vi "Document My VI - Describe My VI.vi"(8 "error in (no error)":errorcluster, 9 "Config Data":cluster{"Company":string, "Author":string}={"Company"="Good Automation, LLC", "Author"="Your Name Here"}, 11 "Active VI Ref In":refnum<vi>) -> (0 "error out":errorcluster, 3 "Active VI Ref Out":refnum<vi>)   [LabVIEW 2014]
uses:
  TYPE_Version Status.ctl
  TYPE_Description Cluster.ctl
  <vilib>/Utility/miscctls.llb/LVBoundsTypeDef.ctl
  <vilib>/regexp/Match Regular Expression.xnode
panel:
  in  "Requirement Coverage":string[](array[string])
  in  "Bold Text":bool
  in  "Copy Desc":bool
  in  "VI Description":string caption="Enter The Text To Provide A Functional Description Of The VI"
  in  "Cancel Button":bool
  out "VI's New Description":string
  out "Icon":picture
  in  "Set No Review":bool
  in  "Use Today":bool
  in  "Date of Review":timestamp=timestamp(3345454800 s since 1904-01-01) format="%<%m/%d/%Y>T"
  in  "Index":u32=1 min=1
  in  "Minor":u16 caption="Major"
  in  "Major":u16 min=1
  in  "Status":T1
  out "Copyright":string
  out "Author(s)":string
  out "VI's Original Description":string
  in  "Save":bool
  # "."
  # "."
  # "Functional Description"
  # "Version Information"
  # "Autoset Information"
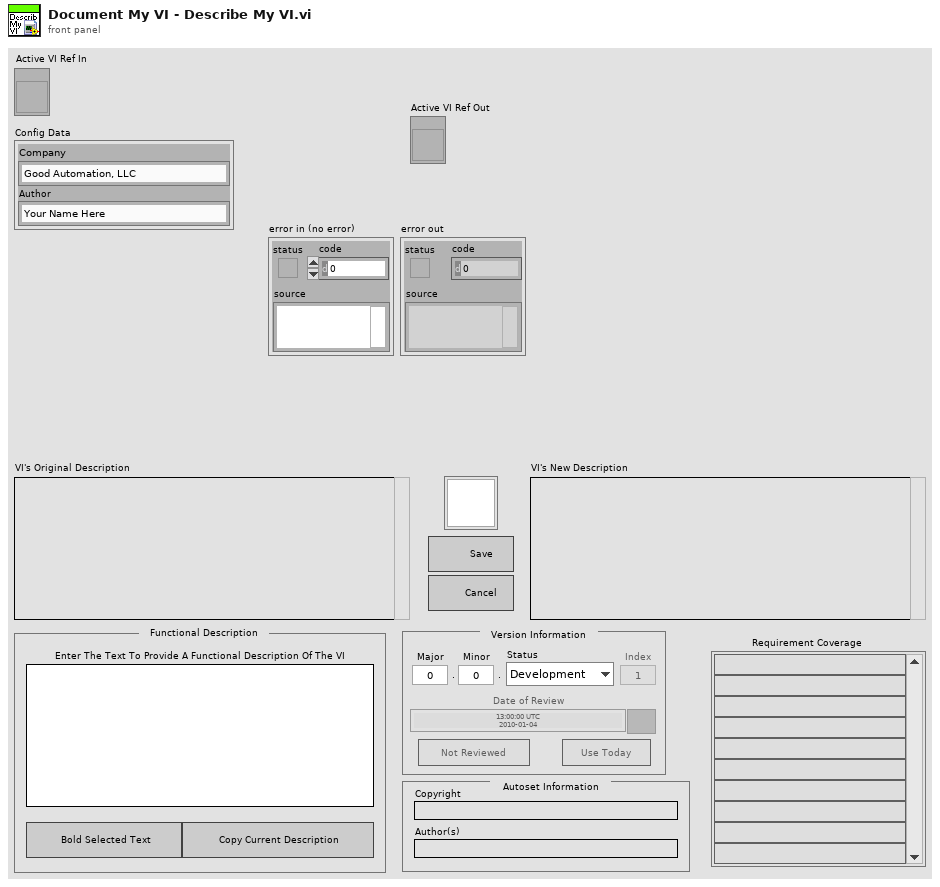
[diagram p1: front panel]
types:
  T1 = typedef "TYPE_Version Status.ctl" = enum16{"Development", "alpha", "beta", "Reviewed", "Bug", "Other"}
  T2 = enum32{"invalid app kind", "Development System", "Run Time System", "Student Edition", "Embedded LabVIEW", "Evaluation", "Custom"}
  T3 = enum8{"Enabled", "Disabled", "Disabled and Grayed Out"}
  T4 = enum32{"Invalid", "Standard", "Closed", "Hidden", "Minimized", "Maximized"}
  T5 = typedef "LVBoundsTypeDef.ctl" = cluster{"Width":u32, "Height":u32}
  T6 = typedef "TYPE_Description Cluster.ctl" = cluster{"VI Description":string, "VI Version":string, "Review Date":string, "Author":string, "Copyright":string, "Requirements Coverage":string}
  T7 = cluster{"Core":cluster{"Current VI Reference":refnum<vi>, "Close Panel on Exit?":bool}, "Config Data":cluster{"Company":string, "Author":string}, "Active VI Ref In":refnum<vi>, "Description":T6, "Original Description":string}
  T8 = cluster{"Current VI Reference":refnum<vi>, "Close Panel on Exit?":bool}
  T9 = typedef "imagedata.ctl" = cluster{"image type":i32, "image depth":i32, "image":u8[], "mask":u8[], "colors":u32[], "Rectangle":cluster{"left":i16, "top":i16, "right":i16, "bottom":i16}}
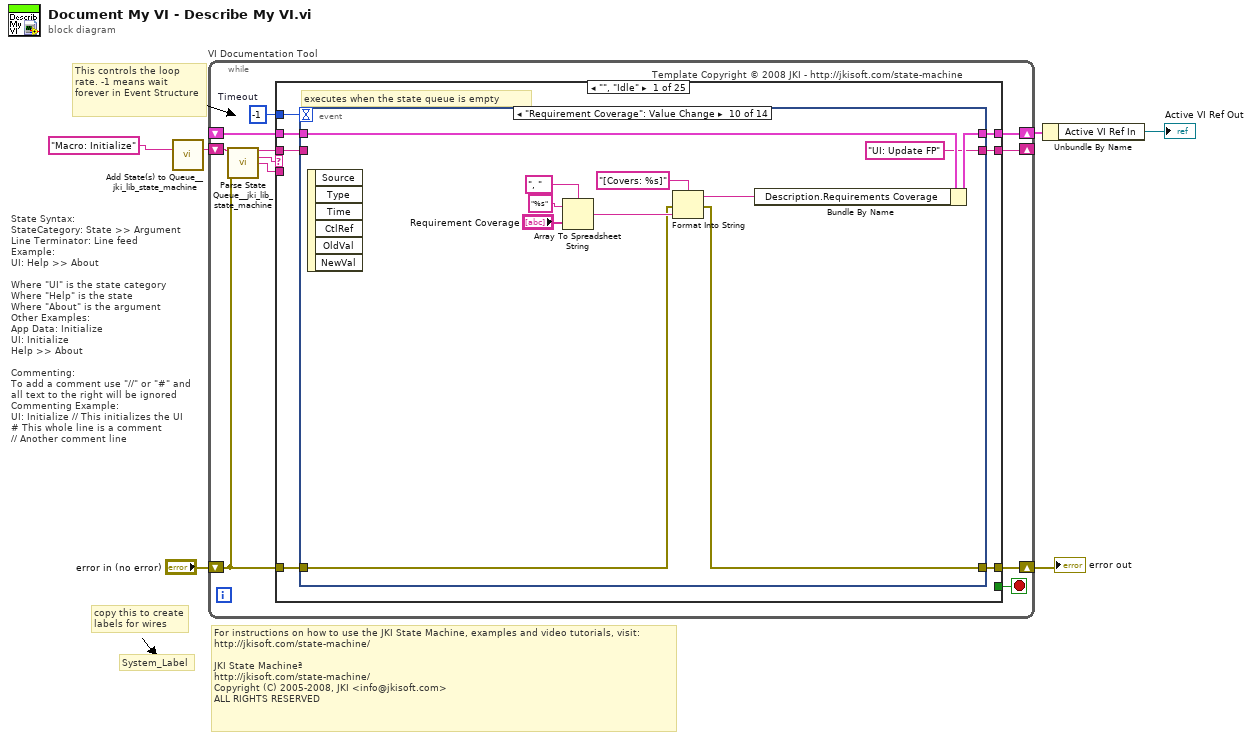
[diagram p0: block diagram]
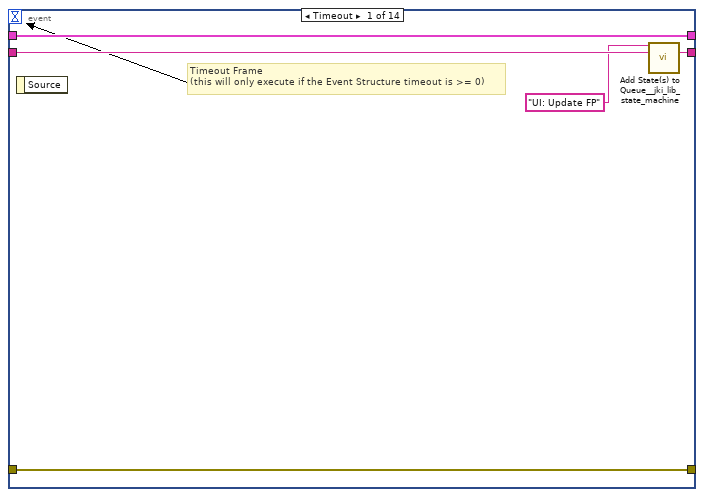
[diagram p2: hidden frame]
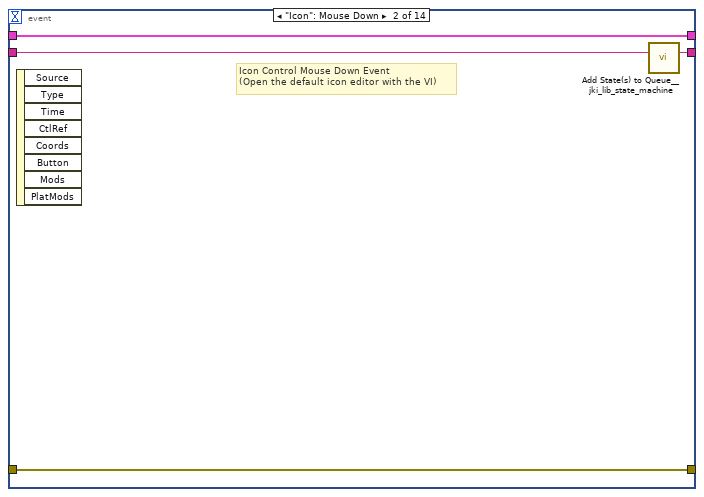
[diagram p3: hidden frame]
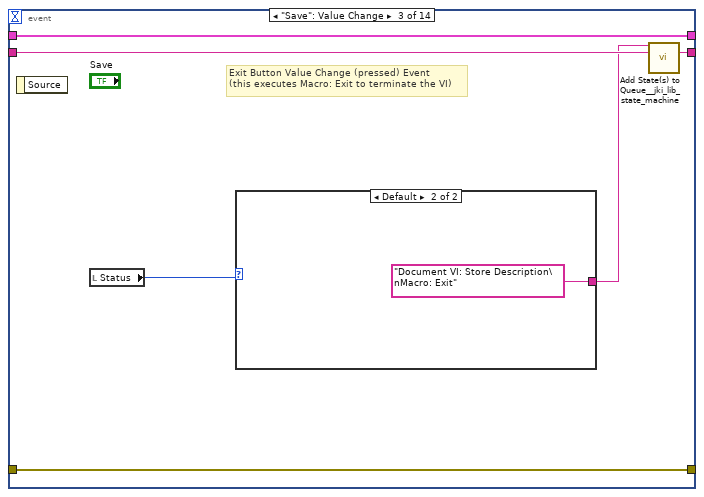
[diagram p4: hidden frame]
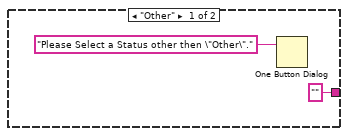
[diagram p5: hidden frame]
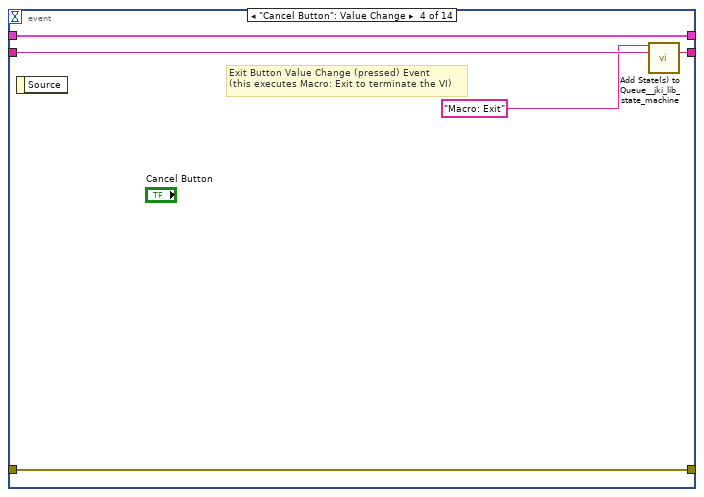
[diagram p6: hidden frame]
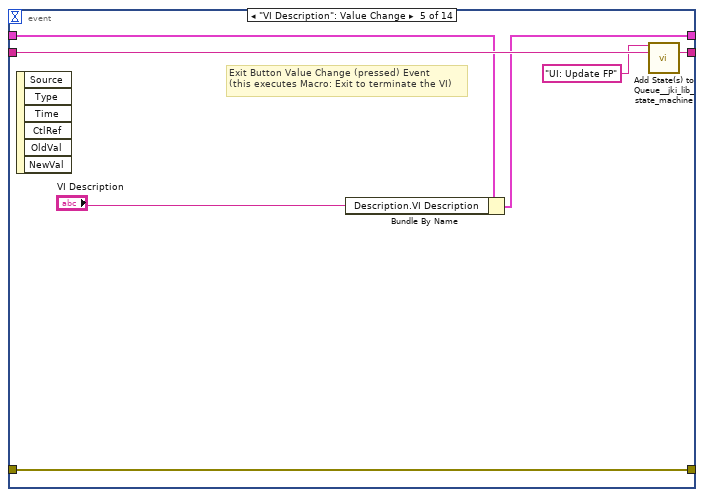
[diagram p7: hidden frame]
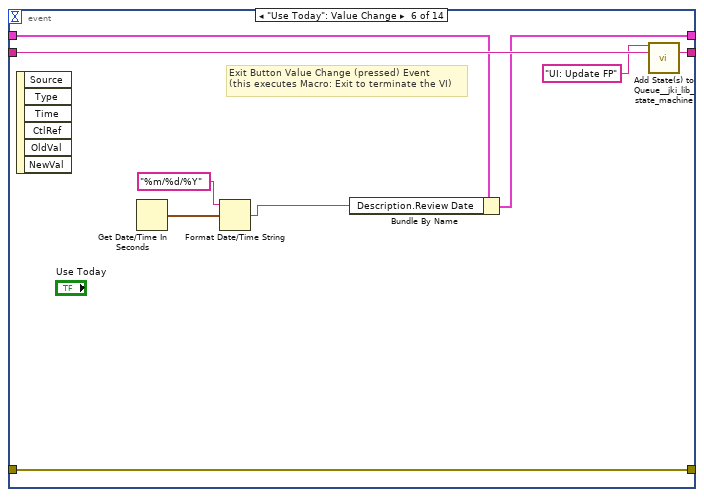
[diagram p8: hidden frame]
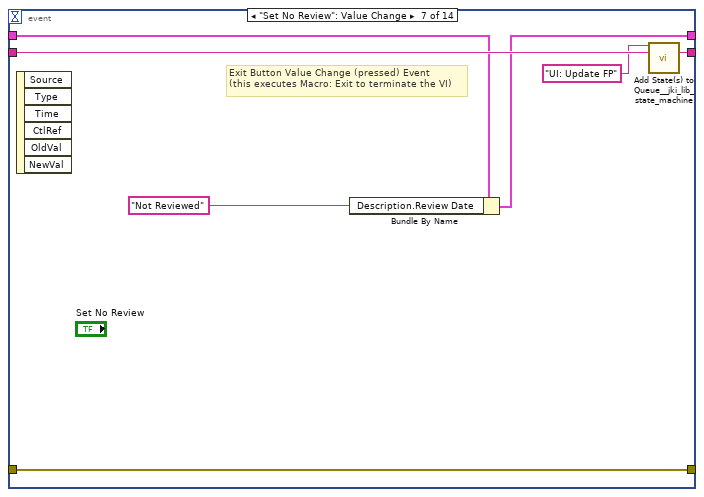
[diagram p9: hidden frame]
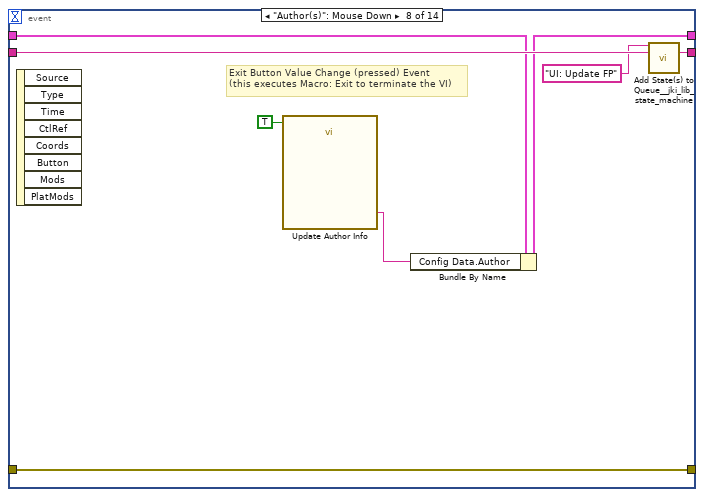
[diagram p10: hidden frame]
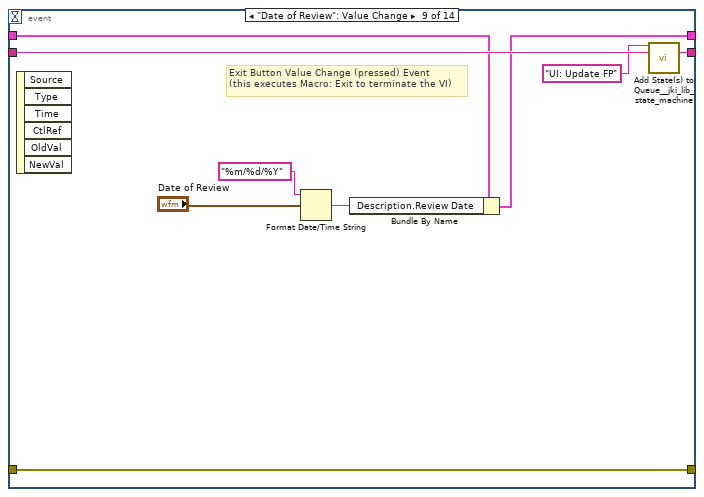
[diagram p11: hidden frame]
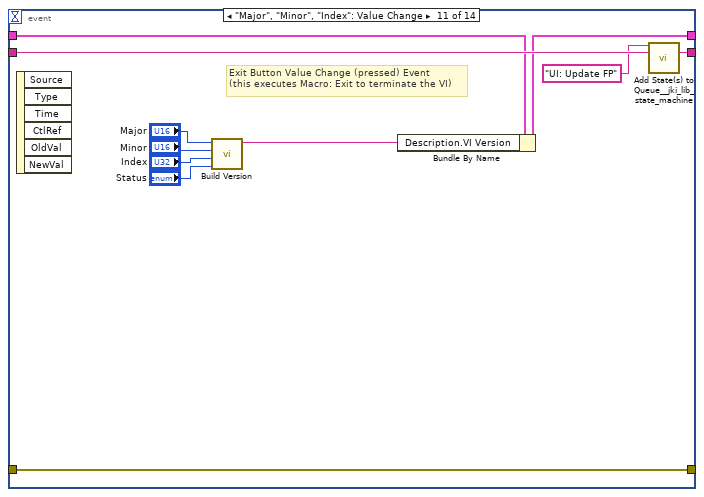
[diagram p12: hidden frame]
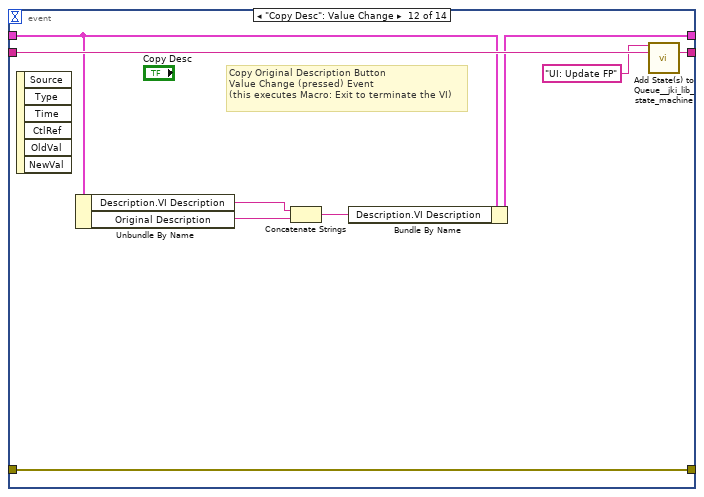
[diagram p13: hidden frame]
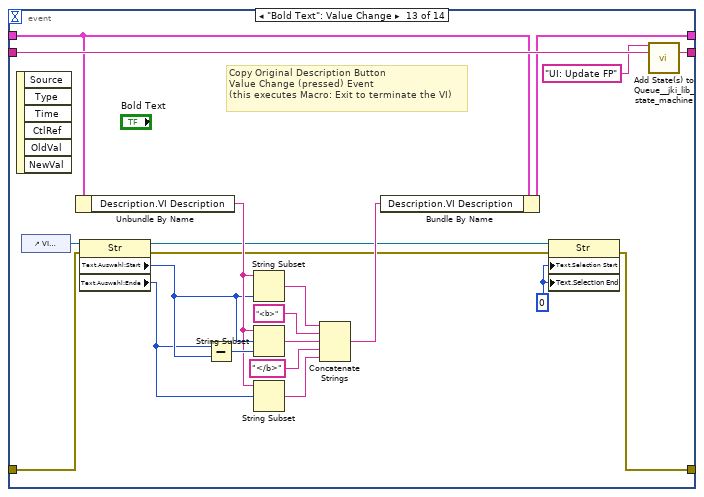
[diagram p14: hidden frame]
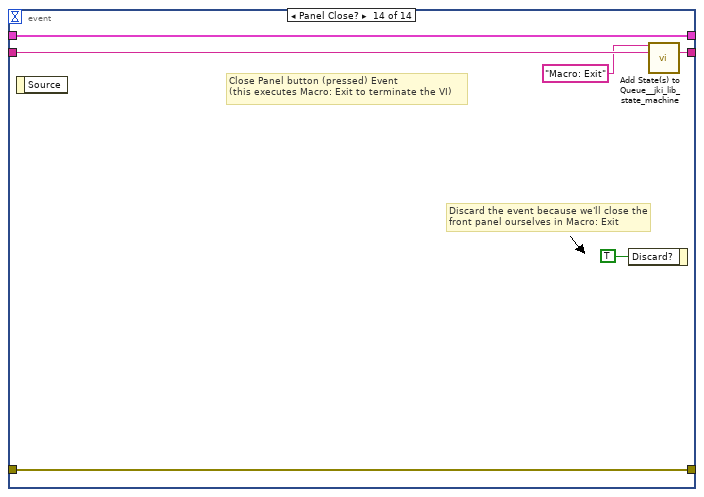
[diagram p15: hidden frame]
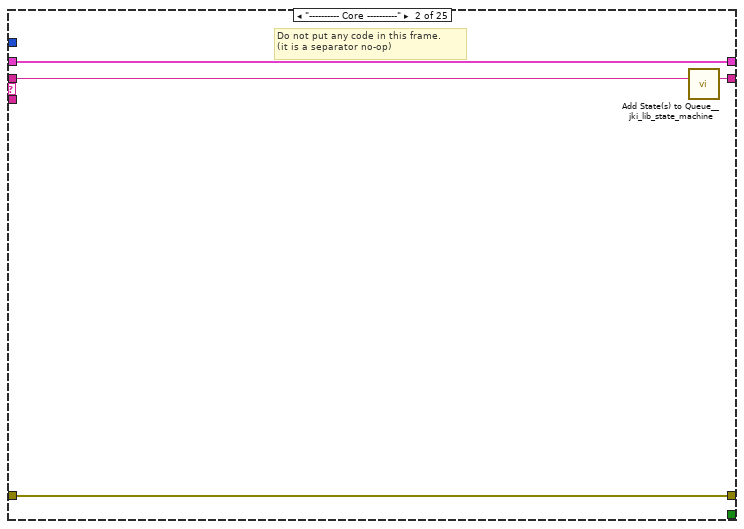
[diagram p16: hidden frame]
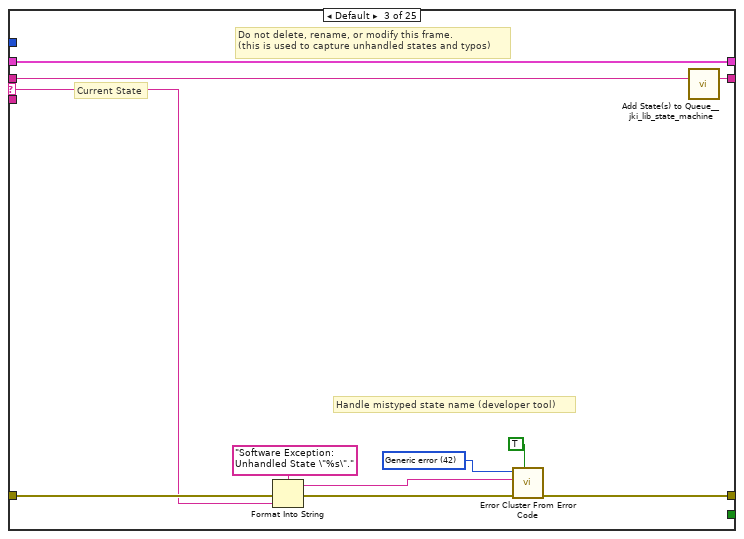
[diagram p17: hidden frame]
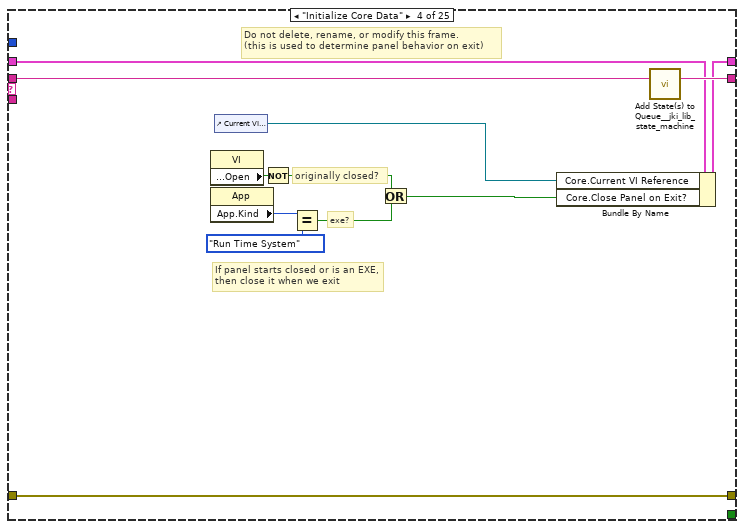
[diagram p18: hidden frame]
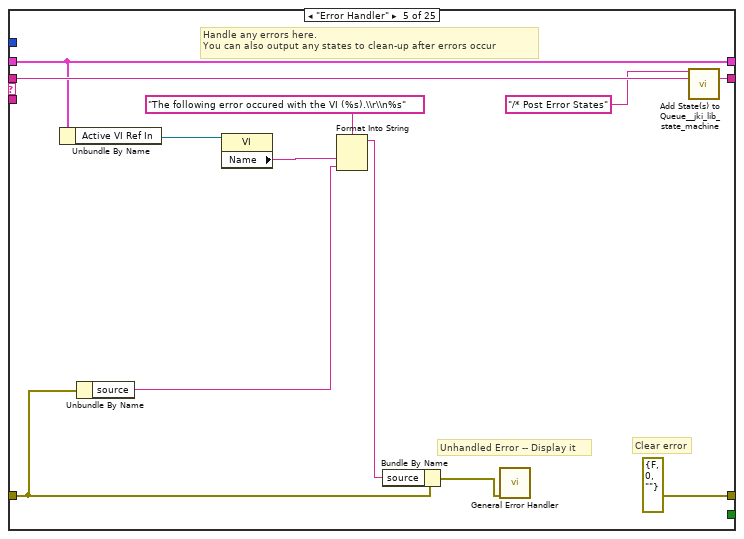
[diagram p19: hidden frame]
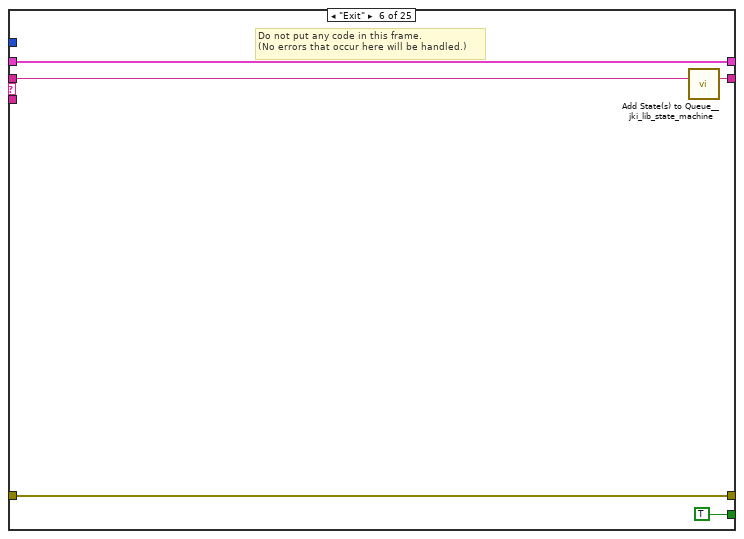
[diagram p20: hidden frame]
diagram:
  # "This controls the loop rate. -1 means wait forever in Event Structure"
  # "For instructions on how to use the JKI State Machine, examples and video tutorials, visit:\nhttp://jkisoft.com/state-machine/\n\nJKI State Machineª\nhttp://jkisoft.com/state-machine/\nCopyright (C) 2005-2008, JKI <info@jkisoft.com>\nALL RIGHTS RESERVED"
  # "State Syntax:\nStateCategory: State >> Argument\nLine Terminator: Line feed\nExample:\nUI: Help >> About\n\nWhere \"UI\" is the state category\nWhere \"Help\" is the state\nWhere \"About\" is the argument\nOther Examples:\nApp Data: Initialize\nUI: Initialize\nHelp >> About\n\nCommenting:\nTo add a comment use \"//\" or \"#\" and all text to the right will be ignored\nCommenting Example:\nUI: Initialize // This initializes the UI\n# This whole line is a comment\n// Another comment line"
  # "copy this to create labels for wires"
  # "System_Label"
  n1 = call <vilib>:"Add State(s) to Queue__jki_lib_state_machine.vi"("State(s) in (\"\")"="Macro: Initialize") -> ("States Out"=w6:string)  [unwired: 14 in]
  n2 = while "VI Documentation Tool" {
    shift-right: [w10] -> w2
    shift-left: _ -> [w9]
    shift-right: [w13] -> w3
    shift-left: "error in (no error)" -> [w7]
    shift-right: [w12] -> _
    shift-left: w6 -> [w14]
    stop <- w11 stop-if-true
    w8 = -1  # Timeout
    # "Template Copyright © 2008 JKI - http://jkisoft.com/state-machine"
    n3 = call <vilib>:"Parse State Queue__jki_lib_state_machine.vi"("State Queue"=w14, "Error In (no error)"=w7) -> ("Remaining States"=w16:string, "Current State"=w17:string, "Arguments"=w15:string)  [unwired: 11 in]
    n4 = case shown="\"\", \"Idle\"" w17 {
      selector: w17 -> [_ _ w150 _ _ _ _ _ _ _ _ _ _ _ _ _ _ _ _ _ _ _ _ _ _]
      tunnel: w16 -> [w24 w149 w154 w172 w184 w189 w193 w202 w208 w212 w218 w245 w372 w393 w404 w430 w435 w445 w450 w455 w459 w475 w489 w504 w517]
      tunnel: w15 -> [_ _ _ _ _ _ _ _ _ _ _ _ _ w388 w398 _ _ _ _ _ _ _ _ _ _]
      tunnel: w9 -> [w22 w146 w152 w163 w179 w187 w190 _ w203 w209 w214 w242 w369 w391 w400 w427 w432 w442 w447 w452 w456 w472 w484 w502 w515]
      tunnel: [w21 w147 w156 w169 errorcluster {"status"=FALSE, "code"=0, "source"=""} ("error out") w186 w191 w199 w204 w210 w215 w243 w370 w389 w401 w428 w433 w443 w448 w453 w457 w468 w479 w500 w513] -> w13
      tunnel: w7 -> [w20 w147 w155 w169 w178 w186 w191 w199 w205 w210 w216 w243 w370 w390 w402 w428 w433 w443 w448 w453 w457 w470 w482 w500 w513]
      tunnel: [w23 w148 w153 w171 w183 w188 w192 w201 w207 w211 w217 w244 w371 w392 w403 w429 w434 w444 w449 w454 w458 w474 w488 w503 w516] -> w12
      tunnel: [_ _ _ _ _ TRUE _ _ _ _ _ _ _ _ _ _ _ _ _ _ _ _ _ _ _] -> w11
      tunnel: [w19 w146 w152 w170 w179 w187 w190 w200 w203 w209 w214 w242 w369 w391 w400 w427 w432 w442 w447 w452 w456 w471 w484 w501 w514] -> w10
      tunnel: w8 -> [w18 _ _ _ _ _ _ _ _ _ _ _ _ _ _ _ _ _ _ _ _ _ _ _ _]
      frame "", "Idle" {
        # "executes when the state queue is empty"
        n5 = event shown="[9] \"Requirement Coverage\": Value Change" {
          selector: _ -> [_ _ _ _ _ _ _ _ _ _ _ _ _ _]
          dyn-events: _ -> [_ _ _ _ _ _ _ _ _ _ _ _ _ _]
          timeout: w18 -> [_ _ _ _ _ _ _ _ _ _ _ _ _ _]
          tunnel: w24 -> [w29 w33 w39 w47 w54 w63 w70 w78 w87 _ w109 w118 w139 w145]
          tunnel: [w28 w32 w38 w46 w53 w62 w69 w77 w86 "UI: Update FP" w108 w117 w138 w144] -> w23
          tunnel: w22 -> [w26 w30 w36 w44 w49 w59 w66 w73 w83 w98 w104 w113 w135 w142]
          tunnel: [w27 w31 w37 w45 w52 w61 w68 w76 w85 w88 w107 w116 w119 w143] -> w21
          tunnel: w20 -> [w27 w31 w37 w45 w52 w61 w68 w76 w85 w89 w107 w116 w121 w143]
          tunnel: [w26 w30 w36 w44 w48 w58 w65 w74 w82 w97 w105 w114 w136 w142] -> w19
          event Timeout {
            # "Timeout Frame\n(this will only execute if the Event Structure timeout is >= 0)"
            n6 = event-data() -> ()  [unwired: 1 in, 1 out]
            n7 = call <vilib>:"Add State(s) to Queue__jki_lib_state_machine.vi"("State(s) in Front (\"\")"="UI: Update FP" ("State(s) in Front (\"\")"), "State(s) in (\"\")"=w29) -> ("States Out"=w28:string)  [unwired: 13 in]
          }
          event "Icon": Mouse Down {
            # "Icon Control Mouse Down Event\n(Open the default icon editor with the VI)"
            n8 = event-data() -> ()  [unwired: 1 in, 8 out]
            n9 = call <vilib>:"Add State(s) to Queue__jki_lib_state_machine.vi"("State(s) in (\"\")"=w33) -> ("States Out"=w32:string)  [unwired: 14 in]
          }
          event "Save": Value Change {
            # "Exit Button Value Change (pressed) Event\n(this executes Macro: Exit to terminate the VI)"
            n10 = event-data() -> ()  [unwired: 1 in, 1 out]
            n11 = local read "Status"() -> (w34:T1)
            n12 = case shown="Default" w34 {
              tunnel: ["" "Document VI: Store Description\nMacro: Exit"] -> w35
              frame "Other" {
                n13 = One Button Dialog(message="Please Select a Status other then \"Other\".") -> ()  [unwired: 1 in, 1 out]
              }
              frame Default {
              }
            }
            n14 = call <vilib>:"Add State(s) to Queue__jki_lib_state_machine.vi"("State(s) in Front (\"\")"=w35, "State(s) in (\"\")"=w39) -> ("States Out"=w38:string)  [unwired: 13 in]
          }
          event "Cancel Button": Value Change {
            # "Exit Button Value Change (pressed) Event\n(this executes Macro: Exit to terminate the VI)"
            n15 = event-data() -> ()  [unwired: 1 in, 1 out]
            n16 = call <vilib>:"Add State(s) to Queue__jki_lib_state_machine.vi"("State(s) in Front (\"\")"="Macro: Exit", "State(s) in (\"\")"=w47) -> ("States Out"=w46:string)  [unwired: 13 in]
          }
          event "VI Description": Value Change {
            # "Exit Button Value Change (pressed) Event\n(this executes Macro: Exit to terminate the VI)"
            n17 = event-data() -> ()  [unwired: 1 in, 6 out]
            n18 = Bundle By Name(cluster=w49, "Description.VI Description"="VI Description") -> (w48:T7)
            n19 = call <vilib>:"Add State(s) to Queue__jki_lib_state_machine.vi"("State(s) in Front (\"\")"="UI: Update FP", "State(s) in (\"\")"=w54) -> ("States Out"=w53:string)  [unwired: 13 in]
          }
          event "Use Today": Value Change {
            # "Exit Button Value Change (pressed) Event\n(this executes Macro: Exit to terminate the VI)"
            n20 = event-data() -> ()  [unwired: 1 in, 6 out]
            n21 = Get Date/Time In Seconds() -> (seconds since 1Jan1904=w57:timestamp)
            n22 = Format Date/Time String(time format string (%c)="%m/%d/%Y", seconds (now)=w57) -> (date/time string=w56:string)  [unwired: 1 in]
            n23 = Bundle By Name(cluster=w59, "Description.Review Date"=w56) -> (w58:T7)
            n24 = call <vilib>:"Add State(s) to Queue__jki_lib_state_machine.vi"("State(s) in Front (\"\")"="UI: Update FP", "State(s) in (\"\")"=w63) -> ("States Out"=w62:string)  [unwired: 13 in]
          }
          event "Set No Review": Value Change {
            # "Exit Button Value Change (pressed) Event\n(this executes Macro: Exit to terminate the VI)"
            n25 = event-data() -> ()  [unwired: 1 in, 6 out]
            n26 = Bundle By Name(cluster=w66, "Description.Review Date"="Not Reviewed" ("time format string (%c)")) -> (w65:T7)
            n27 = call <vilib>:"Add State(s) to Queue__jki_lib_state_machine.vi"("State(s) in Front (\"\")"="UI: Update FP", "State(s) in (\"\")"=w70) -> ("States Out"=w69:string)  [unwired: 13 in]
          }
          event "Author(s)": Mouse Down {
            # "Exit Button Value Change (pressed) Event\n(this executes Macro: Exit to terminate the VI)"
            n28 = event-data() -> ()  [unwired: 1 in, 8 out]
            n29 = call "Update Author Info"("Enable"=TRUE) -> ("Author"=w71:string)  [unwired: 16 in, 2 out]
            n30 = Bundle By Name(cluster=w73, "Config Data.Author"=w71) -> (w74:T7)
            n31 = call <vilib>:"Add State(s) to Queue__jki_lib_state_machine.vi"("State(s) in Front (\"\")"="UI: Update FP", "State(s) in (\"\")"=w78) -> ("States Out"=w77:string)  [unwired: 13 in]
          }
          event "Date of Review": Value Change {
            # "Exit Button Value Change (pressed) Event\n(this executes Macro: Exit to terminate the VI)"
            n32 = event-data() -> ()  [unwired: 1 in, 6 out]
            n33 = Format Date/Time String(time format string (%c)="%m/%d/%Y", seconds (now)="Date of Review") -> (date/time string=w80:string)  [unwired: 1 in]
            n34 = Bundle By Name(cluster=w83, "Description.Review Date"=w80) -> (w82:T7)
            n35 = call <vilib>:"Add State(s) to Queue__jki_lib_state_machine.vi"("State(s) in Front (\"\")"="UI: Update FP", "State(s) in (\"\")"=w87) -> ("States Out"=w86:string)  [unwired: 13 in]
          }
          event "Requirement Coverage": Value Change {
            n36 = event-data() -> ()  [unwired: 1 in, 6 out]
            n37 = Array To Spreadsheet String(delimiter (Tab)=", ", array="Requirement Coverage", 3:"%s" ("format string")) -> (spreadsheet string=w94:string)
            n38 = Format Into String(format string="[Covers: %s]", error in=w89, w94) -> (resulting string=w90:string, error out=w88:errorcluster)  [unwired: 1 in]
            n39 = Bundle By Name(cluster=w98, "Description.Requirements Coverage"=w90) -> (w97:T7)
          }
          event "Major", "Minor", "Index": Value Change {
            # "Exit Button Value Change (pressed) Event\n(this executes Macro: Exit to terminate the VI)"
            n40 = event-data() -> ()  [unwired: 1 in, 6 out]
            n41 = call "Build Version.vi"("Current Phase"="Status", "Revision"="Index", "Minor Revision"="Minor", "Major Revision"="Major") -> ("VI Version"=w103:string)  [unwired: 7 in]
            n42 = Bundle By Name(cluster=w104, "Description.VI Version"=w103) -> (w105:T7)
            n43 = call <vilib>:"Add State(s) to Queue__jki_lib_state_machine.vi"("State(s) in Front (\"\")"="UI: Update FP", "State(s) in (\"\")"=w109) -> ("States Out"=w108:string)  [unwired: 13 in]
          }
          event "Copy Desc": Value Change {
            # "Copy Original Description Button \nValue Change (pressed) Event\n(this executes Macro: Exit to terminate the VI)"
            n44 = event-data() -> ()  [unwired: 1 in, 6 out]
            n45 = Unbundle By Name(w113) -> ("Description.VI Description"=w110:string, "Original Description"=w111:string)
            n46 = Concatenate Strings(w110, w111) -> (w112:string)
            n47 = Bundle By Name(cluster=w113, "Description.VI Description"=w112) -> (w114:T7)
            n48 = call <vilib>:"Add State(s) to Queue__jki_lib_state_machine.vi"("State(s) in Front (\"\")"="UI: Update FP", "State(s) in (\"\")"=w118) -> ("States Out"=w117:string)  [unwired: 13 in]
          }
          event "Bold Text": Value Change {
            w134 = u32 0 ("Text.Auswahl:Start")
            # "Copy Original Description Button \nValue Change (pressed) Event\n(this executes Macro: Exit to terminate the VI)"
            n49 = event-data() -> ()  [unwired: 1 in, 6 out]
            n50 = control-ref of="VI Description"() -> (w122:refnum<vi>)
            n51 = Unbundle By Name(w135) -> ("Description.VI Description"=w127:string)
            n52 = property class="Str"(reference=w122, error in=w121) -> (reference out=w123:refnum<vi>, error out=w120:errorcluster, "Text.Auswahl:Start"=w126:u32, "Text.Auswahl:Ende"=w125:u32)
            n53 = Subtract(x=w125, y=w126) -> (x-y=w128:u32)
            n54 = String Subset(string=w127, length (rest)=w126) -> (substring=w129:string)  [unwired: 1 in]
            n55 = String Subset(string=w127, offset (0)=w126, length (rest)=w128) -> (substring=w131:string)
            n56 = String Subset(string=w127, offset (0)=w125) -> (substring=w133:string)  [unwired: 1 in]
            n57 = Concatenate Strings(w129, "<b>", w131, "</b>", w133) -> (w124:string)
            n58 = Bundle By Name(cluster=w135, "Description.VI Description"=w124) -> (w136:T7)
            n59 = property class="Str"(reference=w123, error in=w120, "Text.Selection Start"=w134, "Text.Selection End"=w134) -> (error out=w119:errorcluster)  [unwired: 1 out]
            n60 = call <vilib>:"Add State(s) to Queue__jki_lib_state_machine.vi"("State(s) in Front (\"\")"="UI: Update FP", "State(s) in (\"\")"=w139) -> ("States Out"=w138:string)  [unwired: 13 in]
          }
          event Panel Close? {
            # "Discard the event because we'll close the front panel ourselves in Macro: Exit"
            # "Close Panel button (pressed) Event\n(this executes Macro: Exit to terminate the VI)"
            n61 = event-data() -> ()  [unwired: 1 in, 1 out]
            n62 = event-data("Discard?"=TRUE) -> ()  [unwired: 1 in, 1 out]
            n63 = call <vilib>:"Add State(s) to Queue__jki_lib_state_machine.vi"("State(s) in Front (\"\")"="Macro: Exit", "State(s) in (\"\")"=w145) -> ("States Out"=w144:string)  [unwired: 13 in]
          }
        }
      }
      frame "---------- Core ----------" {
        # "Do not put any code in this frame.\n(it is a separator no-op)"
        n64 = call <vilib>:"Add State(s) to Queue__jki_lib_state_machine.vi"("State(s) in (\"\")"=w149) -> ("States Out"=w148:string)  [unwired: 14 in]
      }
      frame Default {
        w159 = 42 items=["No error", "Argument error", "Memory is full", "Out of zone", "End of file", "File already open", "Generic file I/O error", "File not found", "File permission error", "Disk is full", "Duplicate path", "Too many files open", "System feature not enabled", "Resource file not found", "Cannot add resource", "Resource not found", "Image not found", "Image memory error", "Pen does not exist", "Config type invalid", "Config token not found", "Config parse error", "Config memory error", "Bad external code format", "Bad external code offset", "External code not present", "Null window", "Destroy window error", "Null menu", "Print aborted", "Bad print record", "Print driver error", "Windows error during printing", "Memory error during printing", "Print dialog error", "Generic print error", "Invalid device refnum", "Device not found", "Device parameter error", "Device unit error", "Cannot open device", "Device call aborted", "Generic error", "Cancelled by user", "Object ID too low", "Object ID too high", "Object not in heap", "Unknown heap", "Unknown object (invalid DefProc)", "Unknown object (DefProc not in table)", "Message out of range", "Invalid (null) method", "Unknown message", "Manager call not supported", "Bad address", "Network operation in progress", "Network operation timed out", "Connection is busy", "Network attribute not supported", "Network error", "Address in use", "System out of memory", "Connection aborted", "Connection refused", "Not connected", "Already connected", "Connection closed", "Initialization error (interapplication manager)", "Bad occurrence", "Wait on unbound occurrence handler", "Occurrence queue overflow", "Datalog type conflict", "Unused", "Unrecognized type (interapplication manager)", "Memory corrupt", "Failed to make temporary DLL", "Old CIN version", "Drag socket not found", "Failed to load drop-object", "Failed to register OLE object", "Failed to release OLE object", "Format specifier type mismatch", "Unknown format specifier", "Too few format specifiers", "Too many format specifiers", "Scan failed", "Newer CIN version", "Error converting to variant", "Runtime menu error", "Password tampered", "Variant attribute not found", "Incompatible variant data type", "Event data is not available", "Event Store is not present", "Occurrence is not found", "Event Queue is not created", "Event info is not available", "Refnum passed is NULL", "Error retrieving Class GUID", "Error retrieving CoClass GUID", "Error retrieving TypeLib GUID.", "Bad built application magic bytes.", "Specific driver is different from the specific driver associated with the Logical Name.", "There is no session opened to the class driver.", "Max Error", "MAX - Error with config objects", "MAX - Error loading configuration", "MAX - Group not supported"]
        # "Current State"
        # "Do not delete, rename, or modify this frame.\n(this is used to capture unhandled states and typos)"
        # "Handle mistyped state name (developer tool)"
        n65 = Format Into String(format string="Software Exception: Unhandled State \"%s\"." ("message"), error in=w155, w150) -> (resulting string=w158:string, error out=w157:errorcluster)  [unwired: 1 in]
        n66 = call <vilib>:"Error Cluster From Error Code.vi"("show call chain? (False)"=TRUE, "error in (no error)"=w157, "error message (\"\")"=w158, "error code (0)"=w159) -> ("error out"=w156:errorcluster)  [unwired: 5 in]
        n67 = call <vilib>:"Add State(s) to Queue__jki_lib_state_machine.vi"("State(s) in (\"\")"=w154) -> ("States Out"=w153:string)  [unwired: 14 in]
      }
      frame "Initialize Core Data" {
        # "Do not delete, rename, or modify this frame.\n(this is used to determine panel behavior on exit)"
        # "originally closed?"
        # "exe?"
        # "If panel starts closed or is an EXE, then close it when we exit"
        n68 = property class="VI"() -> ("Front Panel.Open"=w168:bool)  [unwired: 2 in, 2 out]
        n69 = property class="App"() -> ("App.Kind"=w167:T2)  [unwired: 2 in, 2 out]
        n70 = control-ref of="Current VI Reference"() -> (w161:refnum<vi>)
        n71 = Not(x=w168) -> (.not. x?=w165:bool)
        n72 = Equal?(x=w167, y=T2."Run Time System" ("Application:Kind")) -> (x = y?=w164:bool)
        n73 = Or(x=w165, y=w164) -> (x .or. y?=w162:bool)
        n74 = Bundle By Name(cluster=w163, "Core.Current VI Reference"=w161, "Core.Close Panel on Exit?"=w162) -> (w170:T7)
        n75 = call <vilib>:"Add State(s) to Queue__jki_lib_state_machine.vi"("State(s) in (\"\")"=w172) -> ("States Out"=w171:string)  [unwired: 14 in]
      }
      frame "Error Handler" {
        # "Unhandled Error -- Display it"
        # "Handle any errors here.\nYou can also output any states to clean-up after errors occur"
        # "Clear error"
        n76 = Unbundle By Name(w179) -> ("Active VI Ref In"=w177:refnum<vi>)
        n77 = Unbundle By Name(w178) -> ("source"=w175:string)
        n78 = property class="VI"(reference=w177) -> ("Name"=w174:string)  [unwired: 1 in, 2 out]
        n79 = Format Into String(format string="The following error occured with the VI (%s).\\r\\n%s", w174, w175) -> (resulting string=w176:string)  [unwired: 2 in, 1 out]
        n80 = Bundle By Name(cluster=w178, "source"=w176) -> (w180:errorcluster)
        n81 = call <vilib>:"General Error Handler.vi"("error in (no error)"=w180) -> ()  [unwired: 10 in, 5 out]
        n82 = call <vilib>:"Add State(s) to Queue__jki_lib_state_machine.vi"("State(s) in Front (\"\")"="/* Post Error States", "State(s) in (\"\")"=w184) -> ("States Out"=w183:string)  [unwired: 13 in]
      }
      frame "Exit" {
        # "Do not put any code in this frame.\n(No errors that occur here will be handled.)"
        n83 = call <vilib>:"Add State(s) to Queue__jki_lib_state_machine.vi"("State(s) in (\"\")"=w189) -> ("States Out"=w188:string)  [unwired: 14 in]
      }
      frame "---------- Data ----------" {
        # "Do not put any code in this frame.\n(It is a separator no-op. You can make a copy of this frame to create a new Data frame)"
        n84 = call <vilib>:"Add State(s) to Queue__jki_lib_state_machine.vi"("State(s) in (\"\")"=w193) -> ("States Out"=w192:string)  [unwired: 14 in]
      }
      frame "Data: Initialize" {
        w195 = ""  # Original Description
        w197 = T6 {"VI Description"="", "VI Version"="", "Review Date"="", "Author"="", "Copyright"="", "Requirements Coverage"=""}  # Description
        w198 = T8 {"Current VI Reference"=refnum, "Close Panel on Exit?"=FALSE}  # Core
        # "do not delete - used by framework"
        # "Data names and types of shift register data are defined by this bundle."
        # "Initialize the shift-register data, here.\n(data names are defined by what you wire into the bundle function)"
        n85 = Bundle("Core"=w198, "Config Data"="Config Data", "Active VI Ref In"="Active VI Ref In", "Description"=w197, "Original Description"=w195) -> (w200:T7)  [unwired: 1 in]
        n86 = call <vilib>:"Add State(s) to Queue__jki_lib_state_machine.vi"("State(s) in (\"\")"=w202) -> ("States Out"=w201:string)  [unwired: 14 in]
      }
      frame "Data: Cleanup" {
        # "Cleanup any data and references, here.\n(this is called automatically, by the Macro: Exit)"
        n87 = Unbundle By Name(w203) -> ("Core.Current VI Reference"=w206:refnum<vi>)
        n88 = Close Reference(reference=w206, error in (no error)=w205) -> (error out=w204:errorcluster)
        n89 = call <vilib>:"Add State(s) to Queue__jki_lib_state_machine.vi"("State(s) in (\"\")"=w208) -> ("States Out"=w207:string)  [unwired: 14 in]
      }
      frame "---------- UI ----------" {
        # "Do not put any code in this frame.\n(It is a separator no-op. You can make a copy of this frame to create a new UI frame)"
        n90 = call <vilib>:"Add State(s) to Queue__jki_lib_state_machine.vi"("State(s) in (\"\")"=w212) -> ("States Out"=w211:string)  [unwired: 14 in]
      }
      frame "UI: Initialize" {
        # "Initialize the User Interface, here.\n(this is called automatically, by the Macro: Init)"
        n91 = Unbundle By Name(w214) -> ("Core.Current VI Reference"=w213:refnum<vi>)
        n92 = invoke class="VI" method="Default Vals.Reinit All"(reference=w213, error in=w216) -> (error out=w215:errorcluster)  [unwired: 1 in, 2 out]
        n93 = call <vilib>:"Add State(s) to Queue__jki_lib_state_machine.vi"("State(s) in (\"\")"=w218) -> ("States Out"=w217:string)  [unwired: 14 in]
      }
      frame "UI: Update FP" {
        # "Update the displayed values on the User Interface, here.\n(this is called automatically, by the Timeout of the Event Structure in Idle)"
        n94 = Unbundle By Name(w242) -> ("Description"=w233:T6, "Description.VI Description"=w239:string, "Description.VI Version"=w235:string, "Description.Review Date"=w232:string, "Config Data.Author"=→"Author(s)":string, "Description.Copyright"=→"Copyright":string, "Description.Requirements Coverage"=w225:string)
        n95 = call "Convert Cluster To Description.vi"("Description Cluster"=w233) -> ("Description String (empty)"=w219:string)  [unwired: 9 in, 1 out]
        n96 = xnode "Match Regular Expression"("input string"=w225, "regular expression"=":[ \\t]*([^\\]]*)") -> ("whole match"=w226:string)  [unwired: 4 in, 4 out]
        n97 = control-ref of="VI's New Description"() -> (w220:refnum<vi>)
        n98 = String Subset(string=w226, offset (0)=1) -> (substring=w228:string)  [unwired: 1 in]
        n99 = call <vilib>:"Trim Whitespace.vi"("string"=w228) -> ("trimmed string"=w221:string)  [unwired: 1 in]
        n100 = case shown="Default" w232 {
          selector: w232 -> [w360 _]
          tunnel: [w361 w363] -> w234
          frame Default {
            n101 = Scan From String(format string="%<%m/%d/%y>T", input string=w360) -> (output 1=w361:timestamp)  [unwired: 3 in, 3 out]
          }
          frame "", "Not Reviewed" {
            n102 = Get Date/Time In Seconds() -> (seconds since 1Jan1904=w363:timestamp)
          }
        }
        n103 = call "String Text Format by Tag.vi"("String in"=w219, "String Ref in"=w220) -> ()  [unwired: 9 in, 1 out]
        n104 = Spreadsheet String To Array(delimiter (Tab)=", ", format string="%s", spreadsheet string=w221, array type (2D Dbl)=string[] [] ("array")) -> (array=w223:string[])
        n105 = local write "Requirement Coverage"(w223) -> ()
        n106 = property on="VI Description" class="Str"("Value"=w239) -> ()  [unwired: 2 in, 2 out]
        n107 = call "Split Version.vi"("VI Version"=w235) -> ("Current Phase"=w236:T1, "Minor Version"=w237:u16, "Major Version"=w238:u16)  [unwired: 7 in, 1 out]
        n108 = local write "Date of Review"(w234) -> ()
        n109 = local write "Minor"(w237) -> ()
        n110 = local write "Major"(w238) -> ()
        n111 = local write "Status"(w236) -> ()
        n112 = call <vilib>:"Add State(s) to Queue__jki_lib_state_machine.vi"("State(s) in Front (\"\")"="UI: Set Available Options" ("State(s) in Front (\"\")"), "State(s) in (\"\")"=w245) -> ("States Out"=w244:string)  [unwired: 13 in]
      }
      frame "UI: Set Available Options" {
        # "Update the displayed values on the User Interface, here.\n(this is called automatically, by the Timeout of the Event Structure in Idle)"
        n113 = Unbundle By Name(w369) -> ("Description.VI Version"=w368:string)
        n114 = call "Split Version.vi"("VI Version"=w368) -> ("Current Phase"=w367:T1)  [unwired: 7 in, 3 out]
        n115 = case shown="\"alpha\", \"beta\"" w367 {
          tunnel: [w373 w376 w379 w382 w385] -> w366
          tunnel: [FALSE FALSE FALSE FALSE TRUE] -> _
          tunnel: [T3."Disabled and Grayed Out" ("Disabled") T3."Disabled and Grayed Out" ("Disabled") T3."Disabled and Grayed Out" ("Disabled") T3."Disabled and Grayed Out" ("Disabled") T3."Enabled" ("Disabled")] -> _
          tunnel: [w373 w376 w379 w382 w385] -> w365
          tunnel: [w373 w376 w379 w382 w385] -> w364
          frame "Development", Default {
            w373 = T3."Disabled and Grayed Out" ("Disabled")
          }
          frame "alpha", "beta" {
            w376 = T3."Disabled and Grayed Out" ("Disabled")
          }
          frame "Reviewed" {
            w379 = T3."Enabled" ("Disabled")
          }
          frame "Bug" {
            w382 = T3."Disabled and Grayed Out" ("Disabled")
          }
          frame "Other" {
            w385 = T3."Disabled and Grayed Out" ("Disabled")
          }
        }
        n116 = property on="Date of Review" class="AbsTime (strict)"("DisabledEnum"=w366) -> ()  [unwired: 2 in, 2 out]
        n117 = property on="Use Today" class="Bool"("DisabledEnum"=w364) -> ()  [unwired: 2 in, 2 out]
        n118 = property on="Set No Review" class="Bool"("DisabledEnum"=w365) -> ()  [unwired: 2 in, 2 out]
        n119 = call <vilib>:"Add State(s) to Queue__jki_lib_state_machine.vi"("State(s) in (\"\")"=w372) -> ("States Out"=w371:string)  [unwired: 14 in]
      }
      frame "UI: Cursor Set" {
        # "Argument"
        # "Set and Unset Cursor Busy.\n(Usage: \"UI: Cursor Set >> Busy|Idle\")"
        n120 = case shown="\"Idle\", Default" w388 {
          tunnel: w390 -> [w395 w397]
          tunnel: [w394 w396] -> w389
          frame "Idle", Default {
            n121 = call <vilib>:"Unset Busy.vi"("error in (no error)"=w395) -> ("error out"=w394:errorcluster)  [unwired: 10 in]
          }
          frame "Busy" {
            n122 = call <vilib>:"Set Busy.vi"("error in (no error)"=w397) -> ("error out"=w396:errorcluster)  [unwired: 9 in, 1 out]
          }
        }
        n123 = call <vilib>:"Add State(s) to Queue__jki_lib_state_machine.vi"("State(s) in (\"\")"=w393) -> ("States Out"=w392:string)  [unwired: 14 in]
      }
      frame "UI: Front Panel State" {
        # "Argument"
        # "Set Front Panel Open or Closed\n(Usage: \"UI: Front Panel State >> Open|Close\")"
        n124 = Unbundle By Name(w400) -> ("Core.Current VI Reference"=w399:refnum<vi>)
        n125 = case shown="\"Open\", Default" w398 {
          tunnel: w402 -> [w408 w421]
          tunnel: [w410 w422] -> w401
          tunnel: w399 -> [w409 w419]
          frame "Open", Default {
            n126 = property class="VI"(reference=w409, error in=w408) -> (reference out=w406:refnum<vi>, error out=w407:errorcluster, "Front Panel.Open"=w405:bool)
            n127 = case shown="True" w405 {
              tunnel: [w413 w416] -> w410
              tunnel: w407 -> [w412 w416]
              tunnel: w406 -> [w411 _]
              frame False {
                n128 = invoke class="VI" method="FP.Open"(reference=w411, error in=w412, "Activate"=TRUE, "State"=T4."Standard") -> (error out=w413:errorcluster)  [unwired: 1 in, 4 out]
              }
              frame True {
              }
            }
          }
          frame "Close" {
            n129 = property class="VI"(reference=w419, error in=w421) -> (reference out=w418:refnum<vi>, error out=w420:errorcluster, "Front Panel.Open"=w417:bool)
            n130 = case shown="True" w417 {
              tunnel: [w423 w426] -> w422
              tunnel: w420 -> [w423 w425]
              tunnel: w418 -> [_ w424]
              frame False {
              }
              frame True {
                n131 = invoke class="VI" method="FP.Close"(reference=w424, error in=w425) -> (error out=w426:errorcluster)  [unwired: 1 in, 2 out]
              }
            }
          }
        }
        n132 = call <vilib>:"Add State(s) to Queue__jki_lib_state_machine.vi"("State(s) in (\"\")"=w404) -> ("States Out"=w403:string)  [unwired: 14 in]
      }
      frame "---------- Macro ----------" {
        # "Do not put any code in this frame.\n(It is a separator no-op. You can make a copy of this frame to create a new Macro frame)"
        n133 = call <vilib>:"Add State(s) to Queue__jki_lib_state_machine.vi"("State(s) in (\"\")"=w430) -> ("States Out"=w429:string)  [unwired: 14 in]
      }
      frame "Macro: Initialize" {
        # "Initialization Macro\n(This is called once, when the VI starts)"
        n134 = call <vilib>:"Add State(s) to Queue__jki_lib_state_machine.vi"("State(s) in Front (\"\")"="Data: Initialize\nInitialize Core Data\nUI: Initialize\nUI: Front Panel State >> Open\nMacro: Extract Description\nMacro: Update New Description", "State(s) in (\"\")"=w435) -> ("States Out"=w434:string)  [unwired: 13 in]
      }
      frame "Macro: Exit" {
        # "Exit Macro\n(This is called once, when the VI exits)"
        n135 = Unbundle By Name(w442) -> ("Core.Close Panel on Exit?"=w441:bool)
        n136 = Select(t="UI: Front Panel State >> Close", s=w441, f="") -> (s? t:f=w438:string)
        n137 = call <vilib>:"Add State(s) to Queue__jki_lib_state_machine.vi"("State(s) in (\"\")"=w438, "State(s) at Back (\"\")"="Data: Cleanup\nExit") -> ("States Out"=w436:string)  [unwired: 13 in]
        n138 = call <vilib>:"Add State(s) to Queue__jki_lib_state_machine.vi"("State(s) in Front (\"\")"=w436, "State(s) in (\"\")"=w445) -> ("States Out"=w444:string)  [unwired: 13 in]
      }
      frame "Macro: Update New Description" {
        # "Determine the action(s) to take based on the item tag sent from the RCF\n()"
        n139 = call <vilib>:"Add State(s) to Queue__jki_lib_state_machine.vi"("State(s) in Front (\"\")"="Document VI: Set Developer's Name\rDocument VI: Set Copyright\rUI: Update FP" ("spreadsheet string"), "State(s) in (\"\")"=w450) -> ("States Out"=w449:string)  [unwired: 13 in]
      }
      frame "Macro: Extract Description" {
        # "Determine the action(s) to take based on the item tag sent from the RCF\n()"
        n140 = call <vilib>:"Add State(s) to Queue__jki_lib_state_machine.vi"("State(s) in Front (\"\")"="Document VI: Extract Description\nUI: Update FP" ("spreadsheet string"), "State(s) in (\"\")"=w455) -> ("States Out"=w454:string)  [unwired: 13 in]
      }
      frame "---------- Document VI ----------" {
        # "Template Separator\n(You can make a copy of, or modify, this frame)"
        n141 = call <vilib>:"Add State(s) to Queue__jki_lib_state_machine.vi"("State(s) in (\"\")"=w459) -> ("States Out"=w458:string)  [unwired: 14 in]
      }
      frame "Document VI: Extract Description" {
        # "Extract the contents of the VI Description Field\n(The contents of this field can be manually set)"
        n142 = Unbundle By Name(w472) -> ("Active VI Ref In"=w467:refnum<vi>)
        n143 = property class="VI"(reference=w467, error in=w470) -> (error out=w473:errorcluster, "Description"=w460:string, "Hist.Revision"=w462:u32)  [unwired: 1 out]
        n144 = property on="Index" class="DigNum (strict)"("Val(Sgnl)"=w462) -> ()  [unwired: 2 in, 2 out]
        n145 = call "Convert Description To Cluster.vi"("Description String (empty)"=w460, "error in (no error)"=w473) -> ("Description Cluster"=w469:T6, "error out"=w468:errorcluster)  [unwired: 8 in]
        n146 = invoke class="VI" method="VI Icon.Get as Image Data"(reference=w467) -> ("ImageData"=w464:T9)  [unwired: 5 in, 5 out]
        n147 = control-ref of="VI's Original Description"() -> (w461:refnum<vi>)
        n148 = Bundle By Name(cluster=w472, "Description"=w469, "Original Description"=w460) -> (w471:T7)
        n149 = call "String Text Format by Tag.vi"("String in"=w460, "String Ref in"=w461) -> ()  [unwired: 9 in, 1 out]
        n150 = call <vilib>:"Draw Flattened Pixmap.vi"("image data"=w464) -> ("new picture"=→"Icon":picture)  [unwired: 8 in]
        n151 = property on="Icon" class="Pict"("ZoomFactor"=sgl 1.5 ("Zoom Factor"), "Draw Area Size"=T5 {"Width"=48, "Height"=48}) -> ()  [unwired: 2 in, 2 out]
        n152 = call <vilib>:"Add State(s) to Queue__jki_lib_state_machine.vi"("State(s) in (\"\")"=w475) -> ("States Out"=w474:string)  [unwired: 14 in]
      }
      frame "Document VI: Store Description" {
        # "Update the contents of the VI Description Field\n(The VI will be automatically saved during this process)"
        n153 = Unbundle By Name(w484) -> ("Active VI Ref In"=w483:refnum<vi>, "Description"=w485:T6)
        n154 = call "Convert Cluster To Description.vi"("Description Cluster"=w485, "error in (no error)"=w482) -> ("Description String (empty)"=w487:string, "error out"=w486:errorcluster)  [unwired: 8 in]
        n155 = local read "Status"() -> (w478:T1)
        n156 = property class="VI"(reference=w483, error in=w486, "Description"=w487) -> (reference out=w481:refnum<vi>, error out=w480:errorcluster)
        n157 = Equal?(x=TYPE_Version_Status."Reviewed" ("y"), y=w478) -> (x = y?=w476:bool)
        n158 = call "Lock and Save.vi"("error in (no error)"=w480, "Revision Comments?"=w476, "Lock?"=w476, "VI Ref"=w481) -> ("error out"=w479:errorcluster)  [unwired: 6 in, 1 out]
        n159 = call <vilib>:"Add State(s) to Queue__jki_lib_state_machine.vi"("State(s) in (\"\")"=w489) -> ("States Out"=w488:string)  [unwired: 14 in]
      }
      frame "Document VI: Set Developer's Name" {
        # "Set the name of the Developer of this VI \n(The Developer's name must be set in the options dialog for the plugin)"
        n160 = Unbundle By Name(w502) -> ("Description.Author"=w494:string, "Config Data.Author"=w498:string)
        n161 = Empty String/Path?(string/path=w494) -> (empty?=w493:bool)
        n162 = To Lower Case(string=w494) -> (all lower case string=w496:string)
        n163 = To Lower Case(string=w498) -> (all lower case string=w495:string)
        n164 = Select(t="%s" ("format string"), s=w493, f=", %s" ("format string")) -> (s? t:f=w490:string)
        n165 = Match Pattern(string=w496, regular expression=w495) -> (offset past match=w499:i32)  [unwired: 1 in, 3 out]
        n166 = case shown="0.." w499 {
          tunnel: w494 -> [w508 w509]
          tunnel: w498 -> [w507 _]
          tunnel: [w506 w509] -> w497
          tunnel: w490 -> [w505 _]
          frame ..-1 {
            # "The Developer's name was not found in the string."
            n167 = Format Into String(format string=w505, initial string=w508, w507) -> (resulting string=w506:string)  [unwired: 1 in, 1 out]
          }
          frame 0.. {
            # "The Developer's name was found in the string."
          }
        }
        n168 = Bundle By Name(cluster=w502, "Description.Author"=w497) -> (w501:T7)
        n169 = call <vilib>:"Add State(s) to Queue__jki_lib_state_machine.vi"("State(s) in (\"\")"=w504) -> ("States Out"=w503:string)  [unwired: 14 in]
      }
      frame "Document VI: Set Copyright" {
        # "Set the copyright info for thisVI \n(The copyright must be set in the options dialog for the plugin)"
        n170 = Unbundle By Name(w515) -> ("Description.Copyright"=w512:string, "Config Data.Company"=w511:string)
        n171 = call "Set Copyright.vi"("Company Name"=w511, "Current Copyright"=w512) -> ("Updated Copyright"=w510:string)  [unwired: 9 in]
        n172 = Bundle By Name(cluster=w515, "Description.Copyright"=w510) -> (w514:T7)
        n173 = call <vilib>:"Add State(s) to Queue__jki_lib_state_machine.vi"("State(s) in (\"\")"=w517) -> ("States Out"=w516:string)  [unwired: 14 in]
      }
    }
  }
  "error out" <- w3
  n174 = Unbundle By Name(w2) -> ("Active VI Ref In"=→"Active VI Ref Out":refnum<vi>)
